vi "Stimulus.ParseCSVFile.vi"(8 "error in (no error)":errorcluster, 9 "Add DMM Sweep":bool, 10 "DUTs":bool[](array[boolean])=[FALSE, FALSE, FALSE, FALSE, FALSE, FALSE, FALSE, FALSE, FALSE], 11 "Path":path) -> (0 "error out":errorcluster, 2 "NICSVArray":string[][](array[string]), 3 "path":path)   [LabVIEW 2014, in "NIAnalysis.lvlib"]
uses:
  NIAnalysis.lvlib
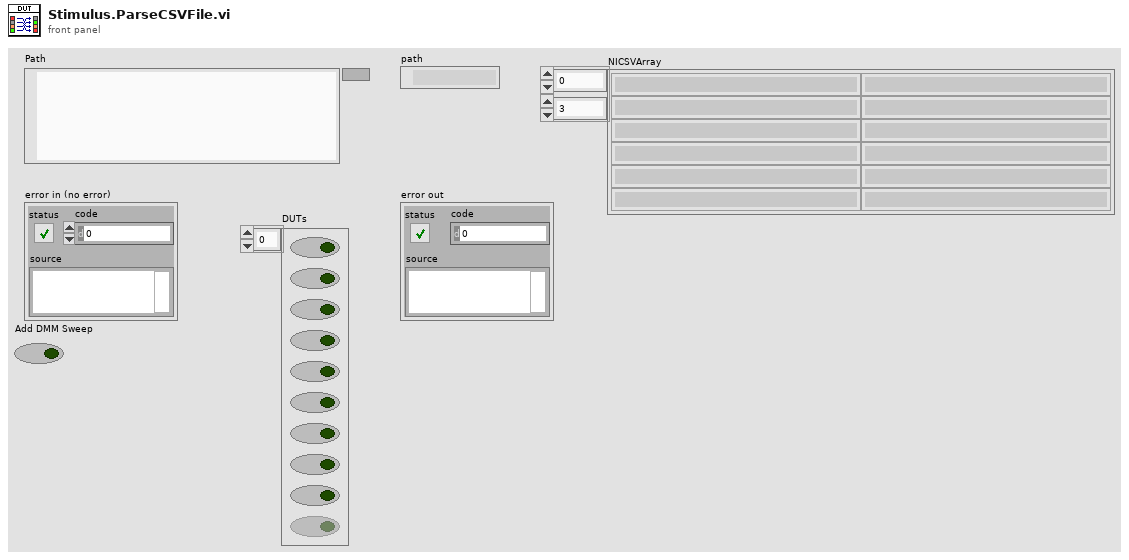
[diagram p1: front panel]
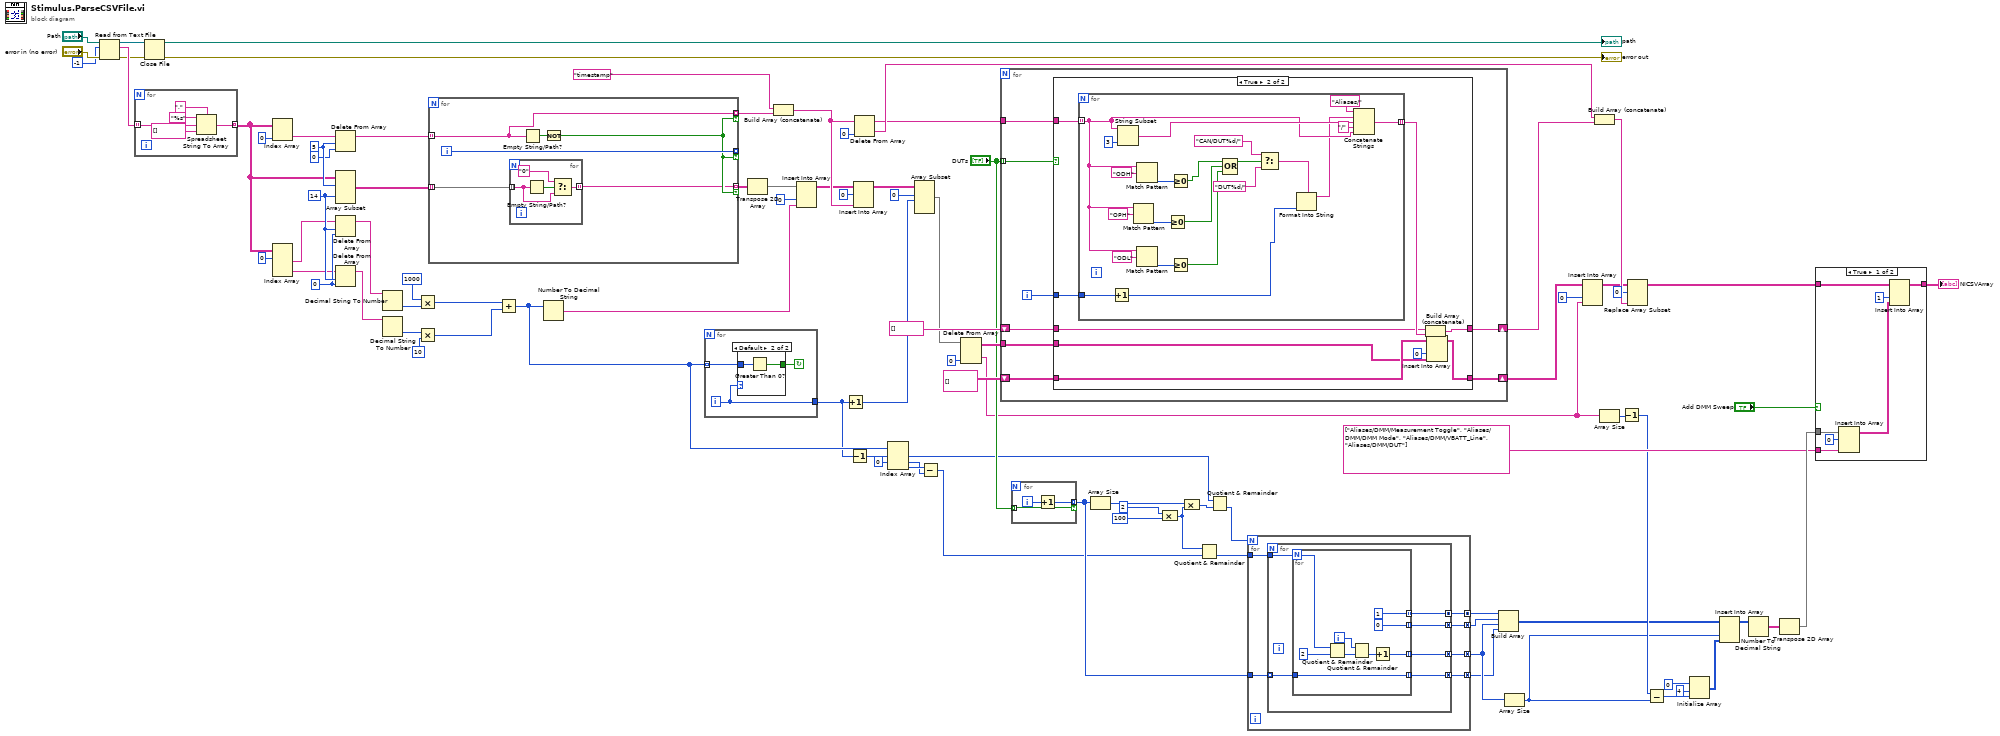
[diagram p0: block diagram]
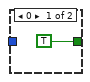
[diagram p4: hidden frame]
diagram:
  w82 = 14 ("index")
  w58 = 0 ("index")
  w81 = 5 ("length")
  n1 = Read from Text File(file (use dialog)="Path", count=-1, error in="error in (no error)") -> (refnum out=w77:refnum<file>, text=w78:string[], error out=w75:errorcluster)  [unwired: 1 in, 1 out]
  n2 = for {
    tunnel: w78 -> [w96] mode=indexing
    tunnel: [w92] -> w68 mode=indexing
    n3 = Spreadsheet String To Array(delimiter (Tab)=",", format string="%s", spreadsheet string=w96, array type (2D Dbl)=string[] []) -> (array=w92:string[])
  }
  n4 = Close File(refnum=w77, error in=w75) -> (path=→"path":path, error out=→"error out":errorcluster)
  n5 = Index Array(array=w68, index (col)=0 ("disabled index (col)")) -> (element=w51:string[])  [unwired: 1 in]
  n6 = Index Array(array=w68, index (row) #1=0 ("index (row)")) -> (element #1=w56:string[], element #2=w57:string[])  [unwired: 3 in]
  n7 = Delete From Array(array=w51, length=w81, index=0) -> (array with subset deleted=w53:string[])  [unwired: 1 out]
  n8 = Array Subset(array=w68, index (row)=w81, index (col)=w82) -> (w85:string[][])  [unwired: 2 in]
  n9 = Delete From Array(array=w56, length=w82, index=w58) -> (array with subset deleted=w60:string[])  [unwired: 1 out]
  n10 = Delete From Array(array=w57, length=w82, index=w58) -> (array with subset deleted=w59:string[])  [unwired: 1 out]
  n11 = Decimal String To Number(string=w60) -> (number=w61:i32[])  [unwired: 2 in, 1 out]
  n12 = Decimal String To Number(string=w59) -> (number=w62:i32[])  [unwired: 2 in, 1 out]
  n13 = Multiply(x=1000, y=w61) -> (x*y=w64:i32[])
  n14 = Multiply(x=w62, y=10) -> (x*y=w65:i32[])
  n15 = for {
    tunnel: w53 -> [w97] mode=indexing
    tunnel: [w100] -> _ mode=indexing if=w99
    tunnel: [w97] -> w54 mode=indexing if=w99
    tunnel: w85 -> [w101] mode=indexing
    tunnel: [w98] -> w69 mode=indexing if=w99
    i -> [w100]
    n16 = for {
      tunnel: w101 -> [w105] mode=indexing
      tunnel: [w103] -> w98 mode=indexing
      n17 = Empty String/Path?(string/path=w105) -> (empty?=w106:bool)
      n18 = Select(t="0", s=w106, f=w105) -> (s? t:f=w103:string)
    }
    n19 = Empty String/Path?(string/path=w97) -> (empty?=w102:bool)
    n20 = Not(x=w102) -> (.not. x?=w99:bool)
  }
  n21 = Add(x=w64, y=w65) -> (x+y=w38:i32[])
  n22 = Number To Decimal String(number=w38) -> (decimal integer string=w70:string[])  [unwired: 1 in]
  n23 = for {
    tunnel: w38 -> [w109] mode=indexing
    tunnel: [w107] -> w32
    i -> [w107]
    stop <- w108 continue-if-true
    n24 = case shown="Default" w107 {
      tunnel: w109 -> [_ w112]
      tunnel: [TRUE w111] -> w108
      frame 0 {
      }
      frame Default {
        n25 = Greater Than 0?(x=w112) -> (x > 0?=w111:bool)
      }
    }
  }
  n26 = Transpose 2D Array(2D array=w69) -> (transposed array=w74:string[][])
  n27 = Build Array (concatenate)("timestamp" ("string"), w54) -> (w87:string[])
  n28 = Insert Into Array(array=w74, index (col)=0 ("disabled index (col)"), new element=w70) -> (w72:string[][])  [unwired: 1 in]
  n29 = Increment(x=w32) -> (x+1=w37:i32)
  n30 = Decrement(x=w32) -> (x-1=w31:i32)
  n31 = Insert Into Array(array=w72, index (row)=0, new element=w87) -> (w84:string[][])  [unwired: 1 in]
  n32 = Delete From Array(array=w87, index=0) -> (deleted portion=w89:string, array with subset deleted=w39:string[])  [unwired: 1 in]
  n33 = Index Array(array=w38, index #1=w31, index #2=0 ("index")) -> (element #1=w33:i32, element #2=w27:i32, element #3=w28:i32)  [unwired: 1 in]
  n34 = Array Subset(array=w84, index (row)=0 ("index"), length (row)=w37) -> (w47:string[][])  [unwired: 2 in]
  n35 = Subtract(x=w28, y=w27) -> (x-y=w21:i32)
  n36 = Delete From Array(array=w47, index (col)=0 ("disabled index (col)")) -> (deleted portion=w13:string[], array with subset deleted=w40:string[][])  [unwired: 2 in]
  n37 = for {
    tunnel: w39 -> [w120]
    tunnel: "DUTs" -> [w114] mode=indexing
    shift-right: [w118] -> w41
    shift-left: string[] [] -> [w119]
    tunnel: w40 -> [w116]
    shift-right: [w115] -> w44
    shift-left: string[][] [] -> [w117]
    i -> [w113]
    n38 = case shown="True" w114 {
      tunnel: w120 -> [_ w131]
      tunnel: w119 -> [w122 w129]
      tunnel: [w122 w128] -> w118
      tunnel: w117 -> [w121 w127]
      tunnel: w116 -> [_ w124]
      tunnel: [w121 w126] -> w115
      tunnel: w113 -> [_ w125]
      frame False {
      }
      frame True {
        n39 = for {
          tunnel: w131 -> [w138] mode=indexing
          tunnel: [w146] -> w130 mode=indexing
          tunnel: w125 -> [w135]
          n40 = Increment(x=w135) -> (x+1=w134:i32)
          n41 = String Subset(string=w138, length (rest)=3 ("length (rest)")) -> (substring=w148:string)  [unwired: 1 in]
          n42 = Match Pattern(string=w138, regular expression="OPH") -> (offset past match=w152:i32)  [unwired: 1 in, 3 out]
          n43 = Match Pattern(string=w138, regular expression="ODH") -> (offset past match=w144:i32)  [unwired: 1 in, 3 out]
          n44 = Match Pattern(string=w138, regular expression="ODL") -> (offset past match=w140:i32)  [unwired: 1 in, 3 out]
          n45 = Greater Or Equal To 0?(x=w152) -> (x >= 0?=w145:bool)
          n46 = Greater Or Equal To 0?(x=w144) -> (x >= 0?=w141:bool)
          n47 = Greater Or Equal To 0?(x=w140) -> (x >= 0?=w137:bool)
          n48 = Compound Arithmetic op=OR(w141, w145, w137) -> (w142:bool)
          n49 = Select(t="CAN/DUT%d/" ("string"), s=w142, f="DUT%d/" ("string")) -> (s? t:f=w133:string)
          n50 = Format Into String(format string=w133, w134) -> (resulting string=w132:string)  [unwired: 2 in, 1 out]
          n51 = Concatenate Strings("Aliases/" ("string"), w132, w148, "/" ("string"), w138) -> (w146:string)
        }
        n52 = Build Array (concatenate)(w129, w130) -> (w128:string[])
        n53 = Insert Into Array(array=w127, index (col)=0 ("disabled index (col)"), new element=w124) -> (w126:string[][])  [unwired: 1 in]
      }
    }
  }
  n54 = for {
    tunnel: "DUTs" -> [w154] mode=indexing
    tunnel: [w155] -> w25 mode=indexing if=w154
    i -> [w156]
    n55 = Increment(x=w156) -> (x+1=w155:i32)
  }
  n56 = Array Size(array=w25) -> (size(s)=w35:i32)
  n57 = Compound Arithmetic op=MULTIPLY(2 ("y"), 100 ("value")) -> (w22:i32)
  n58 = Compound Arithmetic op=MULTIPLY(w35, w22) -> (w34:i32)
  n59 = Quotient & Remainder(x=w22, y=w21) -> (floor(x/y)=w26:i32)  [unwired: 1 out]
  n60 = Quotient & Remainder(x=w33, y=w34) -> (floor(x/y)=w30:i32)  [unwired: 1 out]
  n61 = for {
    N: w30 -> [_]
    tunnel: w26 -> [w162]
    tunnel: w25 -> [w161]
    tunnel: [w160] -> w2 mode=concatenating
    tunnel: [w159] -> w3 mode=concatenating
    tunnel: [w158] -> w20 mode=concatenating
    tunnel: [w157] -> w19 mode=concatenating
    n62 = for {
      tunnel: w162 -> [w166]
      tunnel: w161 -> [w168] mode=indexing
      tunnel: [w167] -> w160 mode=concatenating
      tunnel: [w165] -> w159 mode=concatenating
      tunnel: [w164] -> w158 mode=concatenating
      tunnel: [w163] -> w157 mode=concatenating
      n63 = for {
        N: w166 -> [w172]
        tunnel: w168 -> [w177]
        tunnel: [w177] -> w167 mode=indexing
        tunnel: [w175] -> w165 mode=indexing
        tunnel: [1 ("y")] -> w164 mode=indexing
        tunnel: [0 ("y")] -> w163 mode=indexing
        i -> [w169]
        n64 = Quotient & Remainder(x=w172, y=2) -> (floor(x/y)=w170:i32)  [unwired: 1 out]
        n65 = Quotient & Remainder(x=w169, y=w170) -> (floor(x/y)=w176:i32)  [unwired: 1 out]
        n66 = Increment(x=w176) -> (x+1=w175:i32)
      }
    }
  }
  n67 = Build Array(w20, w19, w3, w2) -> (w7:i32[][])
  n68 = Array Size(array=w3) -> (size(s)=w6:i32)
  n69 = Insert Into Array(array=w44, index (col)=0 ("index (row)"), new element=w13) -> (w42:string[][])  [unwired: 1 in]
  n70 = Build Array (concatenate)(w89, w41) -> (w90:string[])
  n71 = Array Size(array=w13) -> (size(s)=w12:i32)
  n72 = Decrement(x=w12) -> (x-1=w11:i32)
  n73 = Replace Array Subset(array=w42, new element=w90, index (row)=0) -> (w15:string[][])  [unwired: 1 in]
  n74 = Subtract(x=w11, y=w6) -> (x-y=w9:i32)
  n75 = Initialize Array(0 ("y"), 4 ("dimension size"), w9) -> (w5:i32[][])
  n76 = Insert Into Array(array=w7, index (col)=w6, new element=w5) -> (w4:i32[][])  [unwired: 1 in]
  n77 = Number To Decimal String(number=w4) -> (decimal integer string=w18:string[][])  [unwired: 1 in]
  n78 = Transpose 2D Array(2D array=w18) -> (transposed array=w17:string[][])
  n79 = case shown="True" "Add DMM Sweep" {
    tunnel: w17 -> [w184 _]
    tunnel: string[] ["Aliases/DMM/Measurement Toggle", "Aliases/DMM/DMM Mode", "Aliases/DMM/VBATT_Line", "Aliases/DMM/DUT"] -> [w183 _]
    tunnel: w15 -> [w181 w185]
    tunnel: [w179 w185] -> w14
    frame True {
      n80 = Insert Into Array(array=w184, index (row)=0, new element=w183) -> (w180:string[][])  [unwired: 1 in]
      n81 = Insert Into Array(array=w181, index (col)=1 ("disabled index (col)"), new element=w180) -> (w179:string[][])  [unwired: 1 in]
    }
    frame False {
    }
  }
  "NICSVArray" <- w14
